vi "Array To Matrix - RA2.vi"(1 "Real 2D Array":dbl[][](array[numeric])) -> (0 "Real Matrix":T1)   [LabVIEW 2018, in "NI_Matrix.lvlib"]
doc: "Converts an array to a matrix of elements of the same type as the array elements. Wire data to the <B>Real 2D Array</B> input to determine the polymorphic instance to use or manually select the instance."
uses:
  NI_Matrix.lvlib
  RealMatrix.ctl
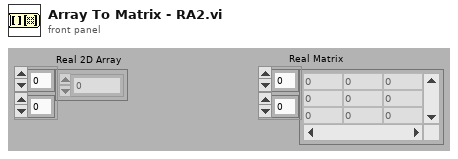
[diagram p1: front panel]
types:
  T1 = typedef "NI_Matrix.lvlib/RealMatrix.ctl" = dbl[][]
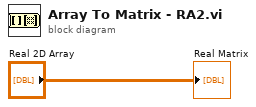
[diagram p0: block diagram]
diagram:
  "Real Matrix" <- "Real 2D Array"
